vi "dvp Vi Get Image Size.vi"(10 "pformat":i32, 11 "handle":u32) -> (2 "pformat out":i32, 3 "function return":u32)   [LabVIEW 2018, in "LabViewDVPCamera.lvlib"]
doc: "LabviewDvp2Api dvpUint32 dvpViGetImageSize(dvpHandle handle, dvpInt32 *pformat);"
uses:
  LabViewDVPCamera.lvlib
  LabViewDVPCamera/LabViewDVPCamera.dll
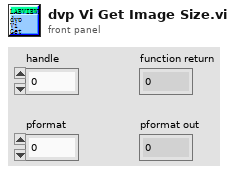
[diagram p1: front panel]
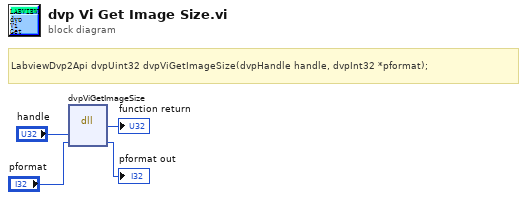
[diagram p0: block diagram]
diagram:
  # "LabviewDvp2Api dvpUint32 dvpViGetImageSize(dvpHandle handle, dvpInt32 *pformat);"
  n1 = dll-call lib="C:/Program Files (x86)/DVP2 Labview cn 64/Sample/LabViewDVPCamera/LabViewDVPCamera.*" fn="dvpViGetImageSize"("handle"="handle", "pformat"="pformat") -> (→"function return":u32, "pformat"=→"pformat out":i32)  [unwired: 4 in, 2 out]
